vi "Stop Scan.vi"(8 "error in (no error)":errorcluster, 11 "PF_API in":refnum<class "PF_API.lvclass">) -> (0 "error out":errorcluster, 3 "PF_API out":refnum<class "PF_API.lvclass">)   [LabVIEW 2019, in "PF_API.lvclass"]
uses:
  PF_API.lvclass
  PF_API.lvclass/PF_API.ctl
  <vilib>/httpClient/POSTBuffer.vi
  <vilib>/httpClient/LabVIEWHTTPClient.lvlib
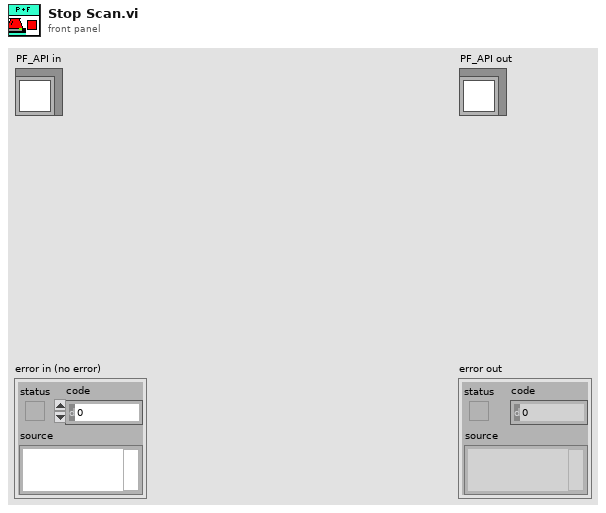
[diagram p1: front panel]
types:
  T1 = typedef "LabVIEWHTTPClient.lvlib/ClientHandle.ctl" = refnum<k1>
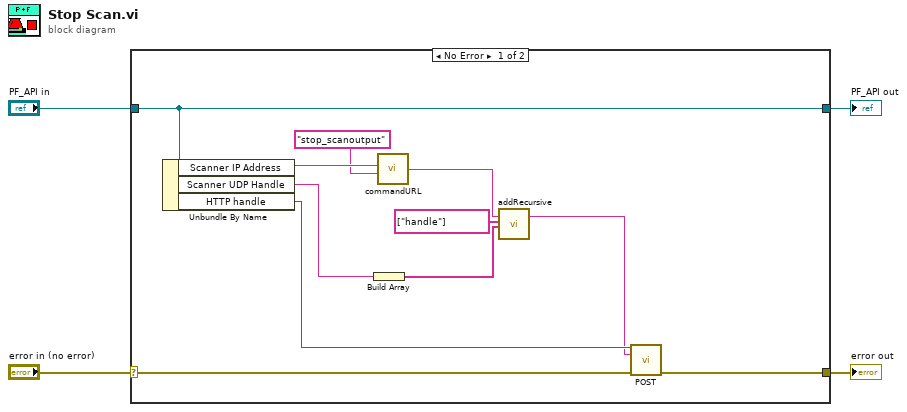
[diagram p0: block diagram]
diagram:
  n1 = case shown="No Error" "error in (no error)" {
    selector: "error in (no error)" -> [w15 w17]
    tunnel: [w7 w17] -> w3
    tunnel: [w14 w16] -> w1
    tunnel: "PF_API in" -> [w14 w16]
    frame No Error {
      n2 = Unbundle By Name(w14) -> ("Scanner IP Address"=w13:string, "Scanner UDP Handle"=w10:string, "HTTP handle"=w6:T1)
      n3 = Build Array(w10) -> (w8:string[])
      n4 = call "commandURL.vi"("Command String"="stop_scanoutput", "Scanner IP Address"=w13) -> ("Command URL"=w11:string)  [unwired: 4 in]
      n5 = call "addRecursive.vi"("Command URL in"=w11, "Parameter Key"=string[] ["handle"], "Parameter Value"=w8) -> ("Command URL out"=w5:string)  [unwired: 13 in, 3 out]
      n6 = call-poly <vilib>:"POST.vi"("client handle"=w6, "url"=w5, "error in (no error)"=w15) -> ("error out"=w7:errorcluster)  [unwired: 9 in, 3 out]
    }
    frame Error {
    }
  }
  "error out" <- w3
  "PF_API out" <- w1
